vi "sub_collect data.vi"(6 "Iteration":i32, 8 "Omega error":errorcluster[](array[cluster]), 9 "Omega task":refnum<k24>[](array[refnum]), 10 "Sensor error":errorcluster, 11 "Sensor task":refnum<k21>) -> (1 "All initialized?":bool, 2 "Elapsed Time (s)":dbl, 3 "Sensor Data":dbl[](array[numeric]))   [LabVIEW 2021]
uses:
  <vilib>/ULx/ULx_LV.dll
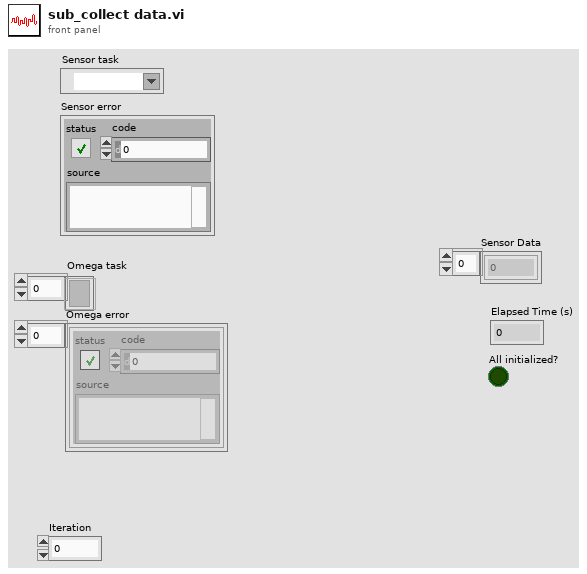
[diagram p1: front panel]
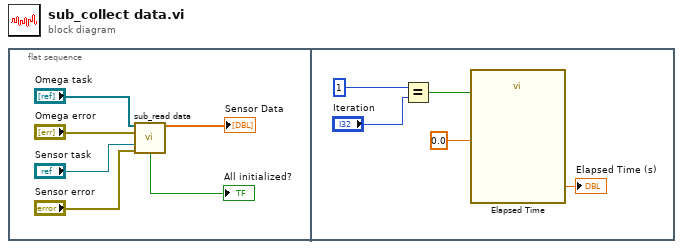
[diagram p0: block diagram]
diagram:
  n1 = flat-sequence {
    frame #0 {
      n2 = call "sub_read data.vi"("Omega task"="Omega task", "Omega error"="Omega error", "Sensor task"="Sensor task", "Sensor error"="Sensor error") -> ("Sensor Data"=→"Sensor Data":dbl[], "All initialized?"=→"All initialized?":bool)  [unwired: 6 in, 4 out]
    }
    frame #1 {
      n3 = Equal?(x=1, y="Iteration") -> (x = y?=w11:bool)
      n4 = call "Elapsed Time"("Reset"=w11, "Set Start Time (s)"=0.0) -> ("Elapsed Time (s)"=→"Elapsed Time (s)":dbl)  [unwired: 10 in, 7 out]
    }
  }
